vi "3 spectraHub- read spectraHub sub.vi"(3 "Goto  wavelength":dbl=402.0, 4 "Integration time(ms)":dbl=1000.0, 5 "XSpectraSense":refnum<k7>(container)) -> (0 "real Wavelength":dbl=401.997 format="%.2f", 1 "SpectraHub output":dbl, 2 "New Integratiom time(ms)":dbl)   [LabVIEW 2011]
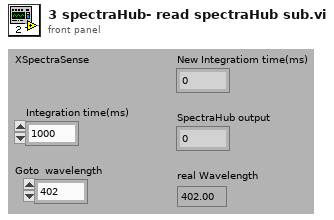
[diagram p1: front panel]
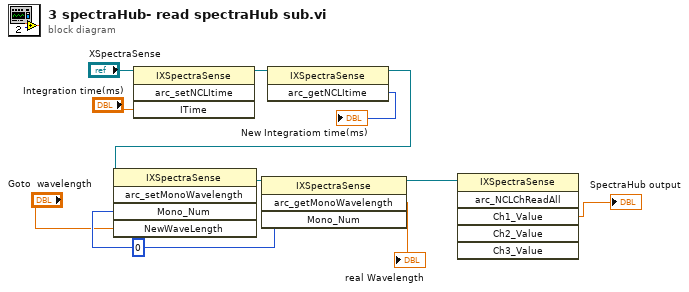
[diagram p0: block diagram]
diagram:
  w8 = 0
  n1 = invoke class="IXSpectraSense" method="arc_setNCLItime"(reference="XSpectraSense", "ITime"="Integration time(ms)") -> (reference out=w1:refnum<k7>)  [unwired: 2 in, 3 out]
  n2 = invoke class="IXSpectraSense" method="arc_getNCLItime"(reference=w1) -> (reference out=w2:refnum<k7>, "arc_getNCLItime"=→"New Integratiom time(ms)":i32)  [unwired: 2 in, 1 out]
  n3 = invoke class="IXSpectraSense" method="arc_setMonoWavelength"(reference=w2, "Mono_Num"=w8, "NewWaveLength"="Goto  wavelength") -> (reference out=w7:refnum<k7>)  [unwired: 2 in, 4 out]
  n4 = invoke class="IXSpectraSense" method="arc_getMonoWavelength"(reference=w7, "Mono_Num"=w8) -> (reference out=w9:refnum<k7>, "arc_getMonoWavelength"=→"real Wavelength":dbl)  [unwired: 2 in, 2 out]
  n5 = invoke class="IXSpectraSense" method="arc_NCLChReadAll"(reference=w9) -> ("Ch1_Value"=→"SpectraHub output":dbl)  [unwired: 5 in, 5 out]
